vi "GeoData.vi"() -> ()   [LabVIEW 2017] (continued)
17051\tVernon\tIL\tFayette County\tH1\n62418\t17051\tBrownstown\tIL\tFayette County\tH1\n62838\t17051\tFarina\tIL\tFayette County\tH1\n62422\t17051\tCowden\tIL\tFayette County\tH1\n62411\t17051\tAltamont\tIL\tFayette County\tH1\n62875\t17051\tPatoka\tIL\tFayette County\tH1\n62431\t17051\tHerrick\tIL\tFayette County\tH1\n62262\t17051\tMulberry grove\tIL\tFayette County\tH1\n62880\t17051\tSaint peter\tIL\tFayette County\tH1\n62080\t17051\tRamsey\tIL\tFayette County\tH1\n62458\t17051\tSaint elmo\tIL\tFayette County\tH1\n62854\t17051\tKinmundy\tIL\tFayette County\tH1\n60921\t17053\tChatsworth\tIL\tFord County\tH1\n61775\t17053\tStrawn\tIL\tFord County\tH1\n60949\t17053\tLudlow\tIL\tFord County\tH1\n60957\t17053\tPaxton\tIL\tFord County\tH1\n60927\t17053\tClifton\tIL\tFord County\tH1\n60929\t17053\tCullom\tIL\tFord County\tH1\n60946\t17053\tKempton\tIL\tFord County\tH1\n60919\t17053\tCabery\tIL\tFord County\tH1\n60918\t17053\tBuckley\tIL\tFord County\tH1\n60959\t17053\tPiper city\tIL\tFord County\tH1\n60941\t17053\tHerscher\tIL\tFord County\tH1\n60936\t17053\tGibson city\tIL\tFord County\tH1\n60968\t17053\tThawville\tIL\tFord County\tH1\n60955\t17053\tOnarga\tIL\tFord County\tH1\n61773\t17053\tSibley\tIL\tFord County\tH1\n60960\t17053\tRankin\tIL\tFord County\tH1\n60933\t17053\tElliott\tIL\tFord County\tH1\n60917\t17053\tBuckingham\tIL\tFord County\tH1\n60948\t17053\tLoda\tIL\tFord County\tH1\n61840\t17053\tDewey\tIL\tFord County\tH1\n61845\t17053\tFoosland\tIL\tFord County\tH1\n61731\t17053\tCropsey\tIL\tFord County\tH1\n60952\t17053\tMelvin\tIL\tFord County\tH1\n60962\t17053\tRoberts\tIL\tFord County\tH1\n62822\t17055\tChristopher\tIL\tFranklin County\tH1\n62999\t17055\tZeigler\tIL\tFranklin County\tH1\n62810\t17055\tBelle rive\tIL\tFranklin County\tH1\n62932\t17055\tElkville\tIL\tFranklin County\tH1\n62812\t17055\tBenton\tIL\tFranklin County\tH1\n62896\t17055\tWest frankfort\tIL\tFranklin County\tH1\n62860\t17055\tMacedonia\tIL\tFranklin County\tH1\n62836\t17055\tEwing\tIL\tFranklin County\tH1\n62983\t17055\tRoyalton\tIL\tFranklin County\tH1\n62897\t17055\tWhittington\tIL\tFranklin County\tH1\n62891\t17055\tValier\tIL\tFranklin County\tH1\n62840\t17055\tFrankfort heights\tIL\tFranklin County\tH1\n62865\t17055\tMulkeytown\tIL\tFranklin County\tH1\n62890\t17055\tThompsonville\tIL\tFranklin County\tH1\n62884\t17055\tSesser\tIL\tFranklin County\tH1\n62883\t17055\tScheller\tIL\tFranklin County\tH1\n62874\t17055\tOrient\tIL\tFranklin County\tH1\n62825\t17055\tCoello\tIL\tFranklin County\tH1\n62819\t17055\tBuckner\tIL\tFranklin County\tH1\n62856\t17055\tLogan\tIL\tFranklin County\tH1\n61531\t17057\tFarmington\tIL\tFulton County\tH1\n61415\t17057\tAvon\tIL\tFulton County\tH1\n61431\t17057\tEllisville\tIL\tFulton County\tH1\n61544\t17057\tLondon mills\tIL\tFulton County\tH1\n61563\t17057\tSaint david\tIL\tFulton County\tH1\n61520\t17057\tCanton\tIL\tFulton County\tH1\n61459\t17057\tMarietta\tIL\tFulton County\tH1\n61432\t17057\tFairview\tIL\tFulton County\tH1\n61542\t17057\tLewistown\tIL\tFulton County\tH1\n61553\t17057\tNorris\tIL\tFulton County\tH1\n61433\t17057\tFiatt\tIL\tFulton County\tH1\n61427\t17057\tCuba\tIL\tFulton County\tH1\n61569\t17057\tTrivoli\tIL\tFulton County\tH1\n61524\t17057\tDunfermline\tIL\tFulton County\tH1\n61477\t17057\tSmithfield\tIL\tFulton County\tH1\n62644\t17057\tHavana\tIL\tFulton County\tH1\n61482\t17057\tTable grove\tIL\tFulton County\tH1\n61484\t17057\tVermont\tIL\tFulton County\tH1\n61533\t17057\tGlasford\tIL\tFulton County\tH1\n61474\t17057\tSaint augustine\tIL\tFulton County\tH1\n61501\t17057\tAstoria\tIL\tFulton County\tH1\n61519\t17057\tBryant\tIL\tFulton County\tH1\n61441\t17057\tIpava\tIL\tFulton County\tH1\n61543\t17057\tLiverpool\tIL\tFulton County\tH1\n62821\t17059\tCarmi\tIL\tGallatin County\tH1\n62867\t17059\tNew haven\tIL\tGallatin County\tH1\n62984\t17059\tShawneetown\tIL\tGallatin County\tH1\n62930\t17059\tEldorado\tIL\tGallatin County\tH1\n62979\t17059\tRidgway\tIL\tGallatin County\tH1\n62934\t17059\tEquality\tIL\tGallatin County\tH1\n62871\t17059\tOmaha\tIL\tGallatin County\tH1\n62869\t17059\tNorris city\tIL\tGallatin County\tH1\n62954\t17059\tJunction\tIL\tGallatin County\tH1\n62027\t17061\tEldred\tIL\tGreene County\tH1\n62092\t17061\tWhite hall\tIL\tGreene County\tH1\n62054\t17061\tKane\tIL\tGreene County\tH1\n62081\t17061\tRockbridge\tIL\tGreene County\tH1\n62050\t17061\tHillview\tIL\tGreene County\tH1\n62078\t17061\tPatterson\tIL\tGreene County\tH1\n62098\t17061\tWrights\tIL\tGreene County\tH1\n62082\t17061\tRoodhouse\tIL\tGreene County\tH1\n62016\t17061\tCarrollton\tIL\tGreene County\tH1\n62044\t17061\tGreenfield\tIL\tGreene County\tH1\n60424\t17063\tGardner\tIL\tGrundy County\tH1\n60481\t17063\tWilmington\tIL\tGrundy County\tH1\n61360\t17063\tSeneca\tIL\tGrundy County\tH1\n60437\t17063\tKinsman\tIL\tGrundy County\tH1\n60470\t17063\tRansom\tIL\tGrundy County\tH1\n60408\t17063\tBraidwood\tIL\tGrundy County\tH1\n60407\t17063\tBraceville\tIL\tGrundy County\tH1\n60474\t17063\tSouth wilmington\tIL\tGrundy County\tH1\n60410\t17063\tChannahon\tIL\tGrundy County\tH1\n60479\t17063\tVerona\tIL\tGrundy County\tH1\n60961\t17063\tReddick\tIL\tGrundy County\tH1\n60447\t17063\tMinooka\tIL\tGrundy County\tH1\n60444\t17063\tMazon\tIL\tGrundy County\tH1\n60416\t17063\tCoal city\tIL\tGrundy County\tH1\n60420\t17063\tDwight\tIL\tGrundy County\tH1\n60541\t17063\tNewark\tIL\tGrundy County\tH1\n60450\t17063\tMorris\tIL\tGrundy County\tH1\n62828\t17065\tDahlgren\tIL\tHamilton County\tH1\n62810\t17065\tBelle rive\tIL\tHamilton County\tH1\n62835\t17065\tEnfield\tIL\tHamilton County\tH1\n62860\t17065\tMacedonia\tIL\tHamilton County\tH1\n62930\t17065\tEldorado\tIL\tHamilton County\tH1\n62817\t17065\tBroughton\tIL\tHamilton County\tH1\n62829\t17065\tDale\tIL\tHamilton County\tH1\n62887\t17065\tSpringerton\tIL\tHamilton County\tH1\n62859\t17065\tMc leansboro\tIL\tHamilton County\tH1\n62935\t17065\tGalatia\tIL\tHamilton County\tH1\n62379\t17067\tWarsaw\tIL\tHancock County\tH1\n62326\t17067\tColchester\tIL\tHancock County\tH1\n62316\t17067\tBowen\tIL\tHancock County\tH1\n62330\t17067\tDallas city\tIL\tHancock County\tH1\n62374\t17067\tTennessee\tIL\tHancock County\tH1\n61450\t17067\tLa harpe\tIL\tHancock County\tH1\n62351\t17067\tMendon\tIL\tHancock County\tH1\n62313\t17067\tBasco\tIL\tHancock County\tH1\n62380\t17067\tWest point\tIL\tHancock County\tH1\n62334\t17067\tElvaston\tIL\tHancock County\tH1\n62341\t17067\tHamilton\tIL\tHancock County\tH1\n62373\t17067\tSutter\tIL\tHancock County\tH1\n62329\t17067\tColusa\tIL\tHancock County\tH1\n61420\t17067\tBlandinsville\tIL\tHancock County\tH1\n62346\t17067\tLa prairie\tIL\tHancock County\tH1\n62321\t17067\tCarthage\tIL\tHancock County\tH1\n62311\t17067\tAugusta\tIL\tHancock County\tH1\n62336\t17067\tFerris\tIL\tHancock County\tH1\n62354\t17067\tNauvoo\tIL\tHancock County\tH1\n62349\t17067\tLoraine\tIL\tHancock County\tH1\n62367\t17067\tPlymouth\tIL\tHancock County\tH1\n62358\t17067\tNiota\tIL\tHancock County\tH1\n62947\t17069\tHerod\tIL\tHardin County\tH1\n62955\t17069\tKarbers ridge\tIL\tHardin County\tH1\n62931\t17069\tElizabethtown\tIL\tHardin County\tH1\n62919\t17069\tCave in rock\tIL\tHardin County\tH1\n62982\t17069\tRosiclare\tIL\tHardin County\tH1\n61418\t17071\tBiggsville\tIL\tHenderson County\tH1\n61460\t17071\tMedia\tIL\tHenderson County\tH1\n62330\t17071\tDallas city\tIL\tHenderson County\tH1\n61454\t17071\tLomax\tIL\tHenderson County\tH1\n61450\t17071\tLa harpe\tIL\tHenderson County\tH1\n61469\t17071\tOquawka\tIL\tHenderson County\tH1\n61471\t17071\tRaritan\tIL\tHenderson County\tH1\n61480\t17071\tStronghurst\tIL\tHenderson County\tH1\n61437\t17071\tGladstone\tIL\tHenderson County\tH1\n61425\t17071\tCarman\tIL\tHenderson County\tH1\n61254\t17073\tGeneseo\tIL\tHenry County\tH1\n61235\t17073\tAtkinson\tIL\tHenry County\tH1\n61233\t17073\tAndover\tIL\tHenry County\tH1\n61240\t17073\tCoal valley\tIL\tHenry County\tH1\n61443\t17073\tKewanee\tIL\tHenry County\tH1\n61344\t17073\tMineral\tIL\tHenry County\tH1\n61241\t17073\tColona\tIL\tHenry County\tH1\n61283\t17073\tTampico\tIL\tHenry County\tH1\n61465\t17073\tNew windsor\tIL\tHenry County\tH1\n61262\t17073\tLynn center\tIL\tHenry County\tH1\n61258\t17073\tHooppole\tIL\tHenry County\tH1\n61238\t17073\tCambridge\tIL\tHenry County\tH1\n61274\t17073\tOsco\tIL\tHenry County\tH1\n61413\t17073\tAlpha\tIL\tHenry County\tH1\n61468\t17073\tOphiem\tIL\tHenry County\tH1\n61490\t17073\tWoodhull\tIL\tHenry County\tH1\n61361\t17073\tSheffield\tIL\tHenry County\tH1\n61419\t17073\tBishop hill\tIL\tHenry County\tH1\n61234\t17073\tAnnawan\tIL\tHenry County\tH1\n61273\t17073\tOrion\tIL\tHenry County\tH1\n61277\t17073\tProphetstown\tIL\tHenry County\tH1\n61250\t17073\tErie\tIL\tHenry County\tH1\n61434\t17073\tGalva\tIL\tHenry County\tH1\n61414\t17073\tAltona\tIL\tHenry County\tH1\n60912\t17075\tBeaverville\tIL\tIroquois County\tH1\n60964\t17075\tSaint anne\tIL\tIroquois County\tH1\n60928\t17075\tCrescent city\tIL\tIroquois County\tH1\n60951\t17075\tMartinton\tIL\tIroquois County\tH1\n60931\t17075\tDonovan\tIL\tIroquois County\tH1\n60939\t17075\tGoodwine\tIL\tIroquois County\tH1\n60927\t17075\tClifton\tIL\tIroquois County\tH1\n60973\t17075\tWellington\tIL\tIroquois County\tH1\n60974\t17075\tWoodland\tIL\tIroquois County\tH1\n60918\t17075\tBuckley\tIL\tIroquois County\tH1\n60956\t17075\tPapineau\tIL\tIroquois County\tH1\n60941\t17075\tHerscher\tIL\tIroquois County\tH1\n60970\t17075\tWatseka\tIL\tIroquois County\tH1\n60966\t17075\tSheldon\tIL\tIroquois County\tH1\n60968\t17075\tThawville\tIL\tIroquois County\tH1\n60955\t17075\tOnarga\tIL\tIroquois County\tH1\n60924\t17075\tCissna park\tIL\tIroquois County\tH1\n60967\t17075\tStockland\tIL\tIroquois County\tH1\n60911\t17075\tAshkum\tIL\tIroquois County\tH1\n60960\t17075\tRankin\tIL\tIroquois County\tH1\n60938\t17075\tGilman\tIL\tIroquois County\tH1\n60953\t17075\tMilford\tIL\tIroquois County\tH1\n60945\t17075\tIroquois\tIL\tIroquois County\tH1\n60926\t17075\tClaytonville\tIL\tIroquois County\tH1\n60930\t17075\tDanforth\tIL\tIroquois County\tH1\n60948\t17075\tLoda\tIL\tIroquois County\tH1\n60942\t17075\tHoopeston\tIL\tIroquois County\tH1\n60922\t17075\tChebanse\tIL\tIroquois County\tH1\n62272\t17077\tPercy\tIL\tJackson County\tH1\n62918\t17077\tCarterville\tIL\tJackson County\tH1\n62975\t17077\tPomona\tIL\tJackson County\tH1\n62932\t17077\tElkville\tIL\tJackson County\tH1\n62942\t17077\tGrand tower\tIL\tJackson County\tH1\n62905\t17077\tAlto pass\tIL\tJackson County\tH1\n62958\t17077\tMakanda\tIL\tJackson County\tH1\n62907\t17077\tAva\tIL\tJackson County\tH1\n62924\t17077\tDe soto\tIL\tJackson County\tH1\n62916\t17077\tCampbell hill\tIL\tJackson County\tH1\n62927\t17077\tDowell\tIL\tJackson County\tH1\n62940\t17077\tGorham\tIL\tJackson County\tH1\n62994\t17077\tVergennes\tIL\tJackson County\tH1\n62950\t17077\tJacob\tIL\tJackson County\tH1\n62901\t17077\tCarbondale\tIL\tJackson County\tH1\n62903\t17077\tCarbondale\tIL\tJackson County\tH1\n62280\t17077\tRockwood\tIL\tJackson County\tH1\n62832\t17077\tDu quoin\tIL\tJackson County\tH1\n62966\t17077\tMurphysboro\tIL\tJackson County\tH1\n62920\t17077\tCobden\tIL\tJackson County\tH1\n62902\t17077\tCarbondale\tIL\tJackson County\tH1\n62448\t17079\tNewton\tIL\tJasper County\tH1\n62479\t17079\tWheeler\tIL\tJasper County\tH1\n62445\t17079\tMontrose\tIL\tJasper County\tH1\n62420\t17079\tCasey\tIL\tJasper County\tH1\n62428\t17079\tGreenup\tIL\tJasper County\tH1\n62425\t17079\tDundas\tIL\tJasper County\tH1\n62481\t17079\tYale\tIL\tJasper County\tH1\n62424\t17079\tDieterich\tIL\tJasper County\tH1\n62432\t17079\tHidalgo\tIL\tJasper County\tH1\n62475\t17079\tWest liberty\tIL\tJasper County\tH1\n62480\t17079\tWillow hill\tIL\tJasper County\tH1\n62436\t17079\tJewett\tIL\tJasper County\tH1\n62459\t17079\tSainte marie\tIL\tJasper County\tH1\n62467\t17079\tTeutopolis\tIL\tJasper County\tH1\n62449\t17079\tOblong\tIL\tJasper County\tH1\n62434\t17079\tIngraham\tIL\tJasper County\tH1\n62864\t17081\tMount vernon\tIL\tJefferson County\tH1\n62872\t17081\tOpdyke\tIL\tJefferson County\tH1\n62828\t17081\tDahlgren\tIL\tJefferson County\tH1\n62810\t17081\tBelle rive\tIL\tJefferson County\tH1\n62851\t17081\tKeenes\tIL\tJefferson County\tH1\n62894\t17081\tWaltonville\tIL\tJefferson County\tH1\n62830\t17081\tDix\tIL\tJefferson County\tH1\n62801\t17081\tCentralia\tIL\tJefferson County\tH1\n62808\t17081\tAshley\tIL\tJefferson County\tH1\n62889\t17081\tTexico\tIL\tJefferson County\tH1\n62860\t17081\tMacedonia\tIL\tJefferson County\tH1\n62816\t17081\tBonnie\tIL\tJefferson County\tH1\n62846\t17081\tIna\tIL\tJefferson County\tH1\n62836\t17081\tEwing\tIL\tJefferson County\tH1\n62893\t17081\tWalnut hill\tIL\tJefferson County\tH1\n62814\t17081\tBluford\tIL\tJefferson County\tH1\n62831\t17081\tDu bois\tIL\tJefferson County\tH1\n62853\t17081\tKell\tIL\tJefferson County\tH1\n62884\t17081\tSesser\tIL\tJefferson County\tH1\n62898\t17081\tWoodlawn\tIL\tJefferson County\tH1\n62883\t17081\tScheller\tIL\tJefferson County\tH1\n62877\t17081\tRichview\tIL\tJefferson County\tH1\n62035\t17083\tGodfrey\tIL\tJersey County\tH1\n62031\t17083\tFieldon\tIL\tJersey County\tH1\n62054\t17083\tKane\tIL\tJersey County\tH1\n62030\t17083\tFidelity\tIL\tJersey County\tH1\n62028\t17083\tElsah\tIL\tJersey County\tH1\n62012\t17083\tBrighton\tIL\tJersey County\tH1\n62052\t17083\tJerseyville\tIL\tJersey County\tH1\n62065\t17083\tMichael\tIL\tJersey County\tH1\n62079\t17083\tPiasa\tIL\tJersey County\tH1\n62037\t17083\tGrafton\tIL\tJersey County\tH1\n62022\t17083\tDow\tIL\tJersey County\tH1\n62063\t17083\tMedora\tIL\tJersey County\tH1\n61085\t17085\tStockton\tIL\tJo Daviess County\tH1\n61036\t17085\tGalena\tIL\tJo Daviess County\tH1\n61053\t17085\tMount carroll\tIL\tJo Daviess County\tH1\n61087\t17085\tWarren\tIL\tJo Daviess County\tH1\n61089\t17085\tWinslow\tIL\tJo Daviess County\tH1\n61062\t17085\tPearl city\tIL\tJo Daviess County\tH1\n61048\t17085\tLena\tIL\tJo Daviess County\tH1\n61044\t17085\tKent\tIL\tJo Daviess County\tH1\n61001\t17085\tApple river\tIL\tJo Daviess County\tH1\n61025\t17085\tEast dubuque\tIL\tJo Daviess County\tH1\n61028\t17085\tElizabeth\tIL\tJo Daviess County\tH1\n61074\t17085\tSavanna\tIL\tJo Daviess County\tH1\n61075\t17085\tScales mound\tIL\tJo Daviess County\tH1\n61059\t17085\tNora\tIL\tJo Daviess County\tH1\n61041\t17085\tHanover\tIL\tJo Daviess County\tH1\n62972\t17087\tOzark\tIL\tJohnson County\tH1\n62985\t17087\tSimpson\tIL\tJohnson County\tH1\n62943\t17087\tGrantsburg\tIL\tJohnson County\tH1\n62938\t17087\tGolconda\tIL\tJohnson County\tH1\n62912\t17087\tBuncombe\tIL\tJohnson County\tH1\n62908\t17087\tBelknap\tIL\tJohnson County\tH1\n62939\t17087\tGoreville\tIL\tJohnson County\tH1\n62922\t17087\tCreal springs\tIL\tJohnson County\tH1\n62909\t17087\tBoles\tIL\tJohnson County\tH1\n62967\t17087\tNew burnside\tIL\tJohnson County\tH1\n62995\t17087\tVienna\tIL\tJohnson County\tH1\n62902\t17087\tCarbondale\tIL\tJohnson County\tH1\n62923\t17087\tCypress\tIL\tJohnson County\tH1\n60136\t17089\tGilberts\tIL\tKane County\tH1\n60144\t17089\tKaneville\tIL\tKane County\tH1\n60192\t17089\tHoffman estates\tIL\tKane County\tH1\n60175\t17089\tSaint charles\tIL\tKane County\tH1\n60502\t17089\tAurora\tIL\tKane County\tH1\n60178\t17089\tSycamore\tIL\tKane County\tH1\n60507\t17089\tAurora\tIL\tKane County\tH1\n60503\t17089\tAurora\tIL\tKane County\tH1\n60103\t17089\tBartlett\tIL\tKane County\tH1\n60110\t17089\tCarpentersville\tIL\tKane County\tH1\n60102\t17089\tAlgonquin\tIL\tKane County\tH1\n60142\t17089\tHuntley\tIL\tKane County\tH1\n60177\t17089\tSouth elgin\tIL\tKane County\tH1\n60123\t17089\tElgin\tIL\tKane County\tH1\n60124\t17089\tElgin\tIL\tKane County\tH1\n60543\t17089\tOswego\tIL\tKane County\tH1\n60538\t17089\tMontgomery\tIL\tKane County\tH1\n60121\t17089\tElgin\tIL\tKane County\tH1\n60184\t17089\tWayne\tIL\tKane County\tH1\n60510\t17089\tBatavia\tIL\tKane County\tH1\n60511\t17089\tBig rock\tIL\tKane County\tH1\n60120\t17089\tElgin\tIL\tKane County\tH1\n60119\t17089\tElburn\tIL\tKane County\tH1\n60542\t17089\tNorth aurora\tIL\tKane County\tH1\n60545\t17089\tPlano\tIL\tKane County\tH1\n60010\t17089\tBarrington\tIL\tKane County\tH1\n60185\t17089\tWest chicago\tIL\tKane County\tH1\n60506\t17089\tAurora\tIL\tKane County\tH1\n60134\t17089\tGeneva\tIL\tKane County\tH1\n60147\t17089\tLafox\tIL\tKane County\tH1\n60520\t17089\tHinckley\tIL\tKane County\tH1\n60135\t17089\tGenoa\tIL\tKane County\tH1\n60109\t17089\tBurlington\tIL\tKane County\tH1\n60183\t17089\tWasco\tIL\tKane County\tH1\n60174\t17089\tSaint charles\tIL\tKane County\tH1\n60504\t17089\tAurora\tIL\tKane County\tH1\n60505\t17089\tAurora\tIL\tKane County\tH1\n60140\t17089\tHampshire\tIL\tKane County\tH1\n60118\t17089\tDundee\tIL\tKane County\tH1\n60151\t17089\tMaple park\tIL\tKane County\tH1\n60554\t17089\tSugar grove\tIL\tKane County\tH1\n60539\t17089\tMooseheart\tIL\tKane County\tH1\n60424\t17091\tGardner\tIL\tKankakee County\tH1\n60481\t17091\tWilmington\tIL\tKankakee County\tH1\n60964\t17091\tSaint anne\tIL\tKankakee County\tH1\n60969\t17091\tUnion hill\tIL\tKankakee County\tH1\n60914\t17091\tBourbonnais\tIL\tKankakee County\tH1\n60954\t17091\tMomence\tIL\tKankakee County\tH1\n60935\t17091\tEssex\tIL\tKankakee County\tH1\n60919\t17091\tCabery\tIL\tKankakee County\tH1\n60401\t17091\tBeecher\tIL\tKankakee County\tH1\n60901\t17091\tKankakee\tIL\tKankakee County\tH1\n60915\t17091\tBradley\tIL\tKankakee County\tH1\n60941\t17091\tHerscher\tIL\tKankakee County\tH1\n60950\t17091\tManteno\tIL\tKankakee County\tH1\n60958\t17091\tPembroke township\tIL\tKankakee County\tH1\n60961\t17091\tReddick\tIL\tKankakee County\tH1\n60944\t17091\tHopkins park\tIL\tKankakee County\tH1\n60910\t17091\tAroma park\tIL\tKankakee County\tH1\n60917\t17091\tBuckingham\tIL\tKankakee County\tH1\n60468\t17091\tPeotone\tIL\tKankakee County\tH1\n60940\t17091\tGrant park\tIL\tKankakee County\tH1\n60922\t17091\tChebanse\tIL\tKankakee County\tH1\n60913\t17091\tBonfield\tIL\tKankakee County\tH1\n60544\t17093\tPlainfield\tIL\tKendall County\tH1\n60548\t17093\tSandwich\tIL\tKendall County\tH1\n60585\t17093\tPlainfield\tIL\tKendall County\tH1\n60431\t17093\tJoliet\tIL\tKendall County\tH1\n60503\t17093\tAurora\tIL\tKendall County\tH1\n60512\t17093\tBristol\tIL\tKendall County\tH1\n60435\t17093\tJoliet\tIL\tKendall County\tH1\n60543\t17093\tOswego\tIL\tKendall County\tH1\n60538\t17093\tMontgomery\tIL\tKendall County\tH1\n60560\t17093\tYorkville\tIL\tKendall County\tH1\n60447\t17093\tMinooka\tIL\tKendall County\tH1\n60511\t17093\tBig rock\tIL\tKendall County\tH1\n60545\t17093\tPlano\tIL\tKendall County\tH1\n60506\t17093\tAurora\tIL\tKendall County\tH1\n60586\t17093\tPlainfield\tIL\tKendall County\tH1\n60541\t17093\tNewark\tIL\tKendall County\tH1\n60536\t17093\tMillbrook\tIL\tKendall County\tH1\n60537\t17093\tMillington\tIL\tKendall County\tH1\n60551\t17093\tSheridan\tIL\tKendall County\tH1\n60450\t17093\tMorris\tIL\tKendall County\tH1\n60504\t17093\tAurora\tIL\tKendall County\tH1\n60554\t17093\tSugar grove\tIL\tKendall County\tH1\n61412\t17095\tAlexis\tIL\tKnox County\tH1\n61529\t17095\tElmwood\tIL\tKnox County\tH1\n61531\t17095\tFarmington\tIL\tKnox County\tH1\n61458\t17095\tMaquon\tIL\tKnox County\tH1\n61449\t17095\tLa fayette\tIL\tKnox County\tH1\n61544\t17095\tLondon mills\tIL\tKnox County\tH1\n61448\t17095\tKnoxville\tIL\tKnox County\tH1\n61410\t17095\tAbingdon\tIL\tKnox County\tH1\n61467\t17095\tOneida\tIL\tKnox County\tH1\n61423\t17095\tCameron\tIL\tKnox County\tH1\n61439\t17095\tHenderson\tIL\tKnox County\tH1\n61401\t17095\tGalesburg\tIL\tKnox County\tH1\n61472\t17095\tRio\tIL\tKnox County\tH1\n61428\t17095\tDahinda\tIL\tKnox County\tH1\n61485\t17095\tVictoria\tIL\tKnox County\tH1\n61490\t17095\tWoodhull\tIL\tKnox County\tH1\n61466\t17095\tNorth henderson\tIL\tKnox County\tH1\n61488\t17095\tWataga\tIL\tKnox County\tH1\n61572\t17095\tYates city\tIL\tKnox County\tH1\n61430\t17095\tEast galesburg\tIL\tKnox County\tH1\n61434\t17095\tGalva\tIL\tKnox County\tH1\n61414\t17095\tAltona\tIL\tKnox County\tH1\n61474\t17095\tSaint augustine\tIL\tKnox County\tH1\n61489\t17095\tWilliamsfield\tIL\tKnox County\tH1\n61436\t17095\tGilson\tIL\tKnox County\tH1\n61402\t17095\tGalesburg\tIL\tKnox County\tH1\n60051\t17097\tMchenry\tIL\tLake County\tH1\n60067\t17097\tPalatine\tIL\tLake County\tH1\n60047\t17097\tLake zurich\tIL\tLake County\tH1\n60050\t17097\tMchenry\tIL\tLake County\tH1\n60042\t17097\tIsland lake\tIL\tLake County\tH1\n60069\t17097\tLincolnshire\tIL\tLake County\tH1\n60090\t17097\tWheeling\tIL\tLake County\tH1\n60089\t17097\tBuffalo grove\tIL\tLake County\tH1\n60013\t17097\tCary\tIL\tLake County\tH1\n60045\t17097\tLake forest\tIL\tLake County\tH1\n60011\t17097\tBarrington\tIL\tLake County\tH1\n60021\t17097\tFox river grove\tIL\tLake County\tH1\n60037\t17097\tFort sheridan\tIL\tLake County\tH1\n60061\t17097\tVernon hills\tIL\tLake County\tH1\n60079\t17097\tWaukegan\tIL\tLake County\tH1\n60002\t17097\tAntioch\tIL\tLake County\tH1\n60073\t17097\tRound lake\tIL\tLake County\tH1\n60084\t17097\tWauconda\tIL\tLake County\tH1\n60088\t17097\tGreat lakes\tIL\tLake County\tH1\n60060\t17097\tMundelein\tIL\tLake County\tH1\n60096\t17097\tWinthrop harbor\tIL\tLake County\tH1\n60015\t17097\tDeerfield\tIL\tLake County\tH1\n60075\t17097\tRussell\tIL\tLake County\tH1\n60085\t17097\tWaukegan\tIL\tLake County\tH1\n60087\t17097\tWaukegan\tIL\tLake County\tH1\n60081\t17097\tSpring grove\tIL\tLake County\tH1\n60099\t17097\tZion\tIL\tLake County\tH1\n60035\t17097\tHighland park\tIL\tLake County\tH1\n60040\t17097\tHighwood\tIL\tLake County\tH1\n60083\t17097\tWadsworth\tIL\tLake County\tH1\n60010\t17097\tBarrington\tIL\tLake County\tH1\n60031\t17097\tGurnee\tIL\tLake County\tH1\n60044\t17097\tLake bluff\tIL\tLake County\tH1\n60074\t17097\tPalatine\tIL\tLake County\tH1\n60064\t17097\tNorth chicago\tIL\tLake County\tH1\n60020\t17097\tFox lake\tIL\tLake County\tH1\n60030\t17097\tGrayslake\tIL\tLake County\tH1\n60046\t17097\tLake villa\tIL\tLake County\tH1\n60048\t17097\tLibertyville\tIL\tLake County\tH1\n60041\t17097\tIngleside\tIL\tLake County\tH1\n60086\t17097\tNorth chicago\tIL\tLake County\tH1\n61360\t17099\tSeneca\tIL\tLaSalle County\tH1\n60437\t17099\tKinsman\tIL\tLaSalle County\tH1\n60552\t17099\tSomonauk\tIL\tLaSalle County\tH1\n60548\t17099\tSandwich\tIL\tLaSalle County\tH1\n60549\t17099\tSerena\tIL\tLaSalle County\tH1\n61373\t17099\tUtica\tIL\tLaSalle County\tH1\n61311\t17099\tAncona\tIL\tLaSalle County\tH1\n61358\t17099\tRutland\tIL\tLaSalle County\tH1\n60470\t17099\tRansom\tIL\tLaSalle County\tH1\n60531\t17099\tLeland\tIL\tLaSalle County\tH1\n61377\t17099\tWenona\tIL\tLaSalle County\tH1\n61301\t17099\tLa salle\tIL\tLaSalle County\tH1\n61342\t17099\tMendota\tIL\tLaSalle County\tH1\n60557\t17099\tWedron\tIL\tLaSalle County\tH1\n61372\t17099\tTroy grove\tIL\tLaSalle County\tH1\n61354\t17099\tPeru\tIL\tLaSalle County\tH1\n61370\t17099\tTonica\tIL\tLaSalle County\tH1\n61336\t17099\tMagnolia\tIL\tLaSalle County\tH1\n60541\t17099\tNewark\tIL\tLaSalle County\tH1\n61348\t17099\tOglesby\tIL\tLaSalle County\tH1\n61350\t17099\tOttawa\tIL\tLaSalle County\tH1\n61334\t17099\tLostant\tIL\tLaSalle County\tH1\n61333\t17099\tLong point\tIL\tLaSalle County\tH1\n61320\t17099\tDalzell\tIL\tLaSalle County\tH1\n60537\t17099\tMillington\tIL\tLaSalle County\tH1\n60551\t17099\tSheridan\tIL\tLaSalle County\tH1\n61364\t17099\tStreator\tIL\tLaSalle County\tH1\n61325\t17099\tGrand ridge\tIL\tLaSalle County\tH1\n61321\t17099\tDana\tIL\tLaSalle County\tH1\n61332\t17099\tLeonore\tIL\tLaSalle County\tH1\n61316\t17099\tCedar point\tIL\tLaSalle County\tH1\n60518\t17099\tEarlville\tIL\tLaSalle County\tH1\n61341\t17099\tMarseilles\tIL\tLaSalle County\tH1\n61371\t17099\tTriumph\tIL\tLaSalle County\tH1\n62439\t17101\tLawrenceville\tIL\tLawrence County\tH1\n62410\t17101\tAllendale\tIL\tLawrence County\tH1\n62466\t17101\tSumner\tIL\tLawrence County\tH1\n62460\t17101\tSaint francisville\tIL\tLawrence County\tH1\n62427\t17101\tFlat rock\tIL\tLawrence County\tH1\n62417\t17101\tBridgeport\tIL\tLawrence County\tH1\n60553\t17103\tSteward\tIL\tLee County\tH1\n61006\t17103\tAshton\tIL\tLee County\tH1\n61349\t17103\tOhio\tIL\tLee County\tH1\n61318\t17103\tCompton\tIL\tLee County\tH1\n61068\t17103\tRochelle\tIL\tLee County\tH1\n61342\t17103\tMendota\tIL\tLee County\tH1\n61353\t17103\tPaw paw\tIL\tLee County\tH1\n61042\t17103\tHarmon\tIL\tLee County\tH1\n61057\t17103\tNachusa\tIL\tLee County\tH1\n61064\t17103\tPolo\tIL\tLee County\tH1\n61243\t17103\tDeer grove\tIL\tLee County\tH1\n61081\t17103\tSterling\tIL\tLee County\tH1\n61376\t17103\tWalnut\tIL\tLee County\tH1\n61031\t17103\tFranklin grove\tIL\tLee County\tH1\n61331\t17103\tLee center\tIL\tLee County\tH1\n60530\t17103\tLee\tIL\tLee County\tH1\n61378\t17103\tWest brooklyn\tIL\tLee County\tH1\n61367\t17103\tSublette\tIL\tLee County\tH1\n61330\t17103\tLa moille\tIL\tLee County\tH1\n61324\t17103\tEldena\tIL\tLee County\tH1\n61071\t17103\tRock falls\tIL\tLee County\tH1\n61021\t17103\tDixon\tIL\tLee County\tH1\n60518\t17103\tEarlville\tIL\tLee County\tH1\n61310\t17103\tAmboy\tIL\tLee County\tH1\n60921\t17105\tChatsworth\tIL\tLivingston County\tH1\n61744\t17105\tGridley\tIL\tLivingston County\tH1\n61775\t17105\tStrawn\tIL\tLivingston County\tH1\n60929\t17105\tCullom\tIL\tLivingston County\tH1\n61311\t17105\tAncona\tIL\tLivingston County\tH1\n61739\t17105\tFairbury\tIL\tLivingston County\tH1\n60470\t17105\tRansom\tIL\tLivingston County\tH1\n60946\t17105\tKempton\tIL\tLivingston County\tH1\n60919\t17105\tCabery\tIL\tLivingston County\tH1\n60959\t17105\tPiper city\tIL\tLivingston County\tH1\n60460\t17105\tOdell\tIL\tLivingston County\tH1\n60961\t17105\tReddick\tIL\tLivingston County\tH1\n61726\t17105\tChenoa\tIL\tLivingston County\tH1\n61728\t17105\tColfax\tIL\tLivingston County\tH1\n60934\t17105\tEmington\tIL\tLivingston County\tH1\n61319\t17105\tCornell\tIL\tLivingston County\tH1\n61743\t17105\tGraymont\tIL\tLivingston County\tH1\n61313\t17105\tBlackstone\tIL\tLivingston County\tH1\n60420\t17105\tDwight\tIL\tLivingston County\tH1\n60917\t17105\tBuckingham\tIL\tLivingston County\tH1\n61333\t17105\tLong point\tIL\tLivingston County\tH1\n61769\t17105\tSaunemin\tIL\tLivingston County\tH1\n61364\t17105\tStreator\tIL\tLivingston County\tH1\n61764\t17105\tPontiac\tIL\tLivingston County\tH1\n61741\t17105\tForrest\tIL\tLivingston County\tH1\n61740\t17105\tFlanagan\tIL\tLivingston County\tH1\n61731\t17105\tCropsey\tIL\tLivingston County\tH1\n60920\t17105\tCampus\tIL\tLivingston County\tH1\n61760\t17105\tMinonk\tIL\tLivingston County\tH1\n60952\t17105\tMelvin\tIL\tLivingston County\tH1\n60962\t17105\tRoberts\tIL\tLivingston County\tH1\n62634\t17107\tElkhart\tIL\tLogan County\tH1\n61723\t17107\tAtlanta\tIL\tLogan County\tH1\n62518\t17107\tChestnut\tIL\tLogan County\tH1\n62519\t17107\tCornland\tIL\tLogan County\tH1\n62548\t17107\tMount pulaski\tIL\tLogan County\tH1\n62656\t17107\tLincoln\tIL\tLogan County\tH1\n62671\t17107\tNew holland\tIL\tLogan County\tH1\n61754\t17107\tMc lean\tIL\tLogan County\tH1\n62682\t17107\tSan jose\tIL\tLogan County\tH1\n61751\t17107\tLawndale\tIL\tLogan County\tH1\n62635\t17107\tEmden\tIL\tLogan County\tH1\n62693\t17107\tWilliamsville\tIL\tLogan County\tH1\n62613\t17107\tAthens\tIL\tLogan County\tH1\n61749\t17107\tKenney\tIL\tLogan County\tH1\n62666\t17107\tMiddletown\tIL\tLogan County\tH1\n62541\t17107\tLake fork\tIL\tLogan County\tH1\n62543\t17107\tLatham\tIL\tLogan County\tH1\n61721\t17107\tArmington\tIL\tLogan County\tH1\n62512\t17107\tBeason\tIL\tLogan County\tH1\n62643\t17107\tHartsburg\tIL\tLogan County\tH1\n61440\t17109\tIndustry\tIL\tMcDonough County\tH1\n61415\t17109\tAvon\tIL\tMcDonough County\tH1\n61475\t17109\tSciota\tIL\tMcDonough County\tH1\n61452\t17109\tLittleton\tIL\tMcDonough County\tH1\n62326\t17109\tColchester\tIL\tMcDonough County\tH1\n61459\t17109\tMarietta\tIL\tMcDonough County\tH1\n62374\t17109\tTennessee\tIL\tMcDonough County\tH1\n61470\t17109\tPrairie city\tIL\tMcDonough County\tH1\n61450\t17109\tLa harpe\tIL\tMcDonough County\tH1\n61473\t17109\tRoseville\tIL\tMcDonough County\tH1\n61455\t17109\tMacomb\tIL\tMcDonough County\tH1\n61438\t17109\tGood hope\tIL\tMcDonough County\tH1\n61422\t17109\tBushnell\tIL\tMcDonough County\tH1\n61411\t17109\tAdair\tIL\tMcDonough County\tH1\n61420\t17109\tBlandinsville\tIL\tMcDonough County\tH1\n61482\t17109\tTable grove\tIL\tMcDonough County\tH1\n61484\t17109\tVermont\tIL\tMcDonough County\tH1\n62367\t17109\tPlymouth\tIL\tMcDonough County\tH1\n61416\t17109\tBardolph\tIL\tMcDonough County\tH1\n60051\t17111\tMchenry\tIL\tMcHenry County\tH1\n60067\t17111\tPalatine\tIL\tMcHenry County\tH1\n60098\t17111\tWoodstock\tIL\tMcHenry County\tH1\n60050\t17111\tMchenry\tIL\tMcHenry County\tH1\n60042\t17111\tIsland lake\tIL\tMcHenry County\tH1\n60152\t17111\tMarengo\tIL\tMcHenry County\tH1\n61012\t17111\tCapron\tIL\tMcHenry County\tH1\n60013\t17111\tCary\tIL\tMcHenry County\tH1\n60021\t17111\tFox river grove\tIL\tMcHenry County\tH1\n60071\t17111\tRichmond\tIL\tMcHenry County\tH1\n60002\t17111\tAntioch\tIL\tMcHenry County\tH1\n60102\t17111\tAlgonquin\tIL\tMcHenry County\tH1\n60142\t17111\tHuntley\tIL\tMcHenry County\tH1\n60072\t17111\tRingwood\tIL\tMcHenry County\tH1\n61038\t17111\tGarden prairie\tIL\tMcHenry County\tH1\n60097\t17111\tWonder lake\tIL\tMcHenry County\tH1\n60081\t17111\tSpring grove\tIL\tMcHenry County\tH1\n60033\t17111\tHarvard\tIL\tMcHenry County\tH1\n60010\t17111\tBarrington\tIL\tMcHenry County\tH1\n60014\t17111\tCrystal lake\tIL\tMcHenry County\tH1\n60156\t17111\tLake in the hills\tIL\tMcHenry County\tH1\n60039\t17111\tCrystal lake\tIL\tMcHenry County\tH1\n60020\t17111\tFox lake\tIL\tMcHenry County\tH1\n60034\t17111\tHebron\tIL\tMcHenry County\tH1\n60135\t17111\tGenoa\tIL\tMcHenry County\tH1\n60012\t17111\tCrystal lake\tIL\tMcHenry County\tH1\n60140\t17111\tHampshire\tIL\tMcHenry County\tH1\n60180\t17111\tUnion\tIL\tMcHenry County\tH1\n61723\t17113\tAtlanta\tIL\tMcLean County\tH1\n61761\t17113\tNormal\tIL\tMcLean County\tH1\n61744\t17113\tGridley\tIL\tMcLean County\tH1\n61745\t17113\tHeyworth\tIL\tMcLean County\tH1\n61770\t17113\tSaybrook\tIL\tMcLean County\tH1\n61776\t17113\tTowanda\tIL\tMcLean County\tH1\n61799\t17113\tBloomington\tIL\tMcLean County\tH1\n61739\t17113\tFairbury\tIL\tMcLean County\tH1\n61732\t17113\tDanvers\tIL\tMcLean County\tH1\n61772\t17113\tShirley\tIL\tMcLean County\tH1\n61759\t17113\tMinier\tIL\tMcLean County\tH1\n61758\t17113\tMerna\tIL\tMcLean County\tH1\n61737\t17113\tEllsworth\tIL\tMcLean County\tH1\n61774\t17113\tStanford\tIL\tMcLean County\tH1\n61724\t17113\tBellflower\tIL\tMcLean County\tH1\n61843\t17113\tFisher\tIL\tMcLean County\tH1\n61790\t17113\tNormal\tIL\tMcLean County\tH1\n60936\t17113\tGibson city\tIL\tMcLean County\tH1\n61701\t17113\tBloomington\tIL\tMcLean County\tH1\n61726\t17113\tChenoa\tIL\tMcLean County\tH1\n61728\t17113\tColfax\tIL\tMcLean County\tH1\n61754\t17113\tMc lean\tIL\tMcLean County\tH1\n61702\t17113\tBloomington\tIL\tMcLean County\tH1\n61722\t17113\tArrowsmith\tIL\tMcLean County\tH1\n61755\t17113\tMackinaw\tIL\tMcLean County\tH1\n61842\t17113\tFarmer city\tIL\tMcLean County\tH1\n61854\t17113\tMansfield\tIL\tMcLean County\tH1\n61725\t17113\tCarlock\tIL\tMcLean County\tH1\n61748\t17113\tHudson\tIL\tMcLean County\tH1\n61752\t17113\tLe roy\tIL\tMcLean County\tH1\n61753\t17113\tLexington\tIL\tMcLean County\tH1\n61730\t17113\tCooksville\tIL\tMcLean County\tH1\n61729\t17113\tCongerville\tIL\tMcLean County\tH1\n61791\t17113\tBloomington\tIL\tMcLean County\tH1\n61705\t17113\tBloomington\tIL\tMcLean County\tH1\n61720\t17113\tAnchor\tIL\tMcLean County\tH1\n61845\t17113\tFoosland\tIL\tMcLean County\tH1\n61738\t17113\tEl paso\tIL\tMcLean County\tH1\n61721\t17113\tArmington\tIL\tMcLean County\tH1\n61731\t17113\tCropsey\tIL\tMcLean County\tH1\n61704\t17113\tBloomington\tIL\tMcLean County\tH1\n61736\t17113\tDowns\tIL\tMcLean County\tH1\n61709\t17113\tBloomington\tIL\tMcLean County\tH1\n62573\t17115\tWarrensburg\tIL\tMacon County\tH1\n62554\t17115\tOreana\tIL\tMacon County\tH1\n62547\t17115\tMount auburn\tIL\tMacon County\tH1\n62549\t17115\tMt zion\tIL\tMacon County\tH1\n62551\t17115\tNiantic\tIL\tMacon County\tH1\n61756\t17115\tMaroa\tIL\tMacon County\tH1\n61937\t17115\tLovington\tIL\tMacon County\tH1\n62537\t17115\tHarristown\tIL\tMacon County\tH1\n61882\t17115\tWeldon\tIL\tMacon County\tH1\n61914\t17115\tBethany\tIL\tMacon County\tH1\n62526\t17115\tDecatur\tIL\tMacon County\tH1\n62539\t17115\tIlliopolis\tIL\tMacon County\tH1\n61925\t17115\tDalton city\tIL\tMacon County\tH1\n62522\t17115\tDecatur\tIL\tMacon County\tH1\n62501\t17115\tArgenta\tIL\tMacon County\tH1\n62523\t17115\tDecatur\tIL\tMacon County\tH1\n61749\t17115\tKenney\tIL\tMacon County\tH1\n62514\t17115\tBoody\tIL\tMacon County\tH1\n62544\t17115\tMacon\tIL\tMacon County\tH1\n62543\t17115\tLatham\tIL\tMacon County\tH1\n62524\t17115\tDecatur\tIL\tMacon County\tH1\n61818\t17115\tCerro gordo\tIL\tMacon County\tH1\n61830\t17115\tCisco\tIL\tMacon County\tH1\n62521\t17115\tDecatur\tIL\tMacon County\tH1\n62513\t17115\tBlue mound\tIL\tMacon County\tH1\n62535\t17115\tForsyth\tIL\tMacon County\tH1\n62550\t17115\tMoweaqua\tIL\tMacon County\tH1\n62525\t17115\tDecatur\tIL\tMacon County\tH1\n62532\t17115\tElwin\tIL\tMacon County\tH1\n62069\t17117\tMount olive\tIL\tMacoupin County\tH1\n62021\t17117\tDorsey\tIL\tMacoupin County\tH1\n62560\t17117\tRaymond\tIL\tMacoupin County\tH1\n62009\t17117\tBenld\tIL\tMacoupin County\tH1\n62056\t17117\tLitchfield\tIL\tMacoupin County\tH1\n62630\t17117\tChesterfield\tIL\tMacoupin County\tH1\n62685\t17117\tShipman\tIL\tMacoupin County\tH1\n62667\t17117\tModesto\tIL\tMacoupin County\tH1\n62012\t17117\tBrighton\tIL\tMacoupin County\tH1\n62674\t17117\tPalmyra\tIL\tMacoupin County\tH1\n62014\t17117\tBunker hill\tIL\tMacoupin County\tH1\n62626\t17117\tCarlinville\tIL\tMacoupin County\tH1\n62672\t17117\tNilwood\tIL\tMacoupin County\tH1\n62033\t17117\tGillespie\tIL\tMacoupin County\tH1\n62088\t17117\tStaunton\tIL\tMacoupin County\tH1\n62097\t17117\tWorden\tIL\tMacoupin County\tH1\n62082\t17117\tRoodhouse\tIL\tMacoupin County\tH1\n62640\t17117\tGirard\tIL\tMacoupin County\tH1\n62079\t17117\tPiasa\tIL\tMacoupin County\tH1\n62091\t17117\tWalshville\tIL\tMacoupin County\tH1\n62638\t17117\tFranklin\tIL\tMacoupin County\tH1\n62093\t17117\tWilsonville\tIL\tMacoupin County\tH1\n62074\t17117\tNew douglas\tIL\tMacoupin County\tH1\n62649\t17117\tHettick\tIL\tMacoupin County\tH1\n62668\t17117\tMurrayville\tIL\tMacoupin County\tH1\n62002\t17117\tAlton\tIL\tMacoupin County\tH1\n62063\t17117\tMedora\tIL\tMacoupin County\tH1\n62044\t17117\tGreenfield\tIL\tMacoupin County\tH1\n62085\t17117\tSawyerville\tIL\tMacoupin County\tH1\n62572\t17117\tWaggoner\tIL\tMacoupin County\tH1\n62690\t17117\tVirden\tIL\tMacoupin County\tH1\n62023\t17117\tEagarville\tIL\tMacoupin County\tH1\n62035\t17119\tGodfrey\tIL\tMadison County\tH1\n62021\t17119\tDorsey\tIL\tMadison County\tH1\n62010\t17119\tBethalto\tIL\tMadison County\tH1\n62025\t17119\tEdwardsville\tIL\tMadison County\tH1\n62060\t17119\tMadison\tIL\tMadison County\tH1\n62249\t17119\tHighland\tIL\tMadison County\tH1\n62275\t17119\tPocahontas\tIL\tMadison County\tH1\n62254\t17119\tLebanon\tIL\tMadison County\tH1\n62048\t17119\tHartford\tIL\tMadison County\tH1\n62084\t17119\tRoxana\tIL\tMadison County\tH1\n62012\t17119\tBrighton\tIL\tMadison County\tH1\n62062\t17119\tMaryville\tIL\tMadison County\tH1\n62201\t17119\tEast saint louis\tIL\tMadison County\tH1\n62001\t17119\tAlhambra\tIL\tMadison County\tH1\n62269\t17119\tO fallon\tIL\tMadison County\tH1\n62058\t17119\tLivingston\tIL\tMadison County\tH1\n62026\t17119\tEdwardsville\tIL\tMadison County\tH1\n62040\t17119\tGranite city\tIL\tMadison County\tH1\n62087\t17119\tSouth roxana\tIL\tMadison County\tH1\n62234\t17119\tCollinsville\tIL\tMadison County\tH1\n62281\t17119\tSaint jacob\tIL\tMadison County\tH1\n62216\t17119\tAviston\tIL\tMadison County\tH1\n62061\t17119\tMarine\tIL\tMadison County\tH1\n62086\t17119\tSorento\tIL\tMadison County\tH1\n62088\t17119\tStaunton\tIL\tMadison County\tH1\n62090\t17119\tVenice\tIL\tMadison County\tH1\n62097\t17119\tWorden\tIL\tMadison County\tH1\n62067\t17119\tMoro\tIL\tMadison County\tH1\n62018\t17119\tCottage hills\tIL\tMadison County\tH1\n62024\t17119\tEast alton\tIL\tMadison County\tH1\n62074\t17119\tNew douglas\tIL\tMadison County\tH1\n62095\t17119\tWood river\tIL\tMadison County\tH1\n62294\t17119\tTroy\tIL\tMadison County\tH1\n62034\t17119\tGlen carbon\tIL\tMadison County\tH1\n62046\t17119\tHamel\tIL\tMadison County\tH1\n62002\t17119\tAlton\tIL\tMadison County\tH1\n62293\t17119\tTrenton\tIL\tMadison County\tH1\n62273\t17119\tPierron\tIL\tMadison County\tH1\n62885\t17121\tShobonier\tIL\tMarion County\tH1\n62892\t17121\tVernon\tIL\tMarion County\tH1\n62899\t17121\tXenia\tIL\tMarion County\tH1\n62882\t17121\tSandoval\tIL\tMarion County\tH1\n62838\t17121\tFarina\tIL\tMarion County\tH1\n62851\t17121\tKeenes\tIL\tMarion County\tH1\n62250\t17121\tHoffman\tIL\tMarion County\tH1\n62807\t17121\tAlma\tIL\tMarion County\tH1\n62830\t17121\tDix\tIL\tMarion County\tH1\n62801\t17121\tCentralia\tIL\tMarion County\tH1\n62875\t17121\tPatoka\tIL\tMarion County\tH1\n62881\t17121\tSalem\tIL\tMarion County\tH1\n62889\t17121\tTexico\tIL\tMarion County\tH1\n62849\t17121\tIuka\tIL\tMarion County\tH1\n62893\t17121\tWalnut hill\tIL\tMarion County\tH1\n62854\t17121\tKinmundy\tIL\tMarion County\tH1\n62853\t17121\tKell\tIL\tMarion County\tH1\n62870\t17121\tOdin\tIL\tMarion County\tH1\n61523\t17123\tChillicothe\tIL\tMarshall County\tH1\n61560\t17123\tPutnam\tIL\tMarshall County\tH1\n61375\t17123\tVarna\tIL\tMarshall County\tH1\n61421\t17123\tBradford\tIL\tMarshall County\tH1\n61358\t17123\tRutland\tIL\tMarshall County\tH1\n61565\t17123\tSparland\tIL\tMarshall County\tH1\n61570\t17123\tWashburn\tIL\tMarshall County\tH1\n61377\t17123\tWenona\tIL\tMarshall County\tH1\n61369\t17123\tToluca\tIL\tMarshall County\tH1\n61424\t17123\tCamp grove\tIL\tMarshall County\tH1\n61526\t17123\tEdelstein\tIL\tMarshall County\tH1\n61537\t17123\tHenry\tIL\tMarshall County\tH1\n61479\t17123\tSpeer\tIL\tMarshall County\tH1\n61336\t17123\tMagnolia\tIL\tMarshall County\tH1\n61541\t17123\tLa rose\tIL\tMarshall County\tH1\n61540\t17123\tLacon\tIL\tMarshall County\tH1\n61321\t17123\tDana\tIL\tMarshall County\tH1\n61760\t17123\tMinonk\tIL\tMarshall County\tH1\n61546\t17125\tManito\tIL\tMason County\tH1\n62627\t17125\tChandlerville\tIL\tMason County\tH1\n62671\t17125\tNew holland\tIL\tMason County\tH1\n62655\t17125\tKilbourne\tIL\tMason County\tH1\n62664\t17125\tMason city\tIL\tMason County\tH1\n62682\t17125\tSan jose\tIL\tMason County\tH1\n61534\t17125\tGreen valley\tIL\tMason County\tH1\n62617\t17125\tBath\tIL\tMason County\tH1\n62644\t17125\tHavana\tIL\tMason County\tH1\n61567\t17125\tTopeka\tIL\tMason County\tH1\n61532\t17125\tForest city\tIL\tMason County\tH1\n62633\t17125\tEaston\tIL\tMason County\tH1\n62960\t17127\tMetropolis\tIL\tMassac County\tH1\n62956\t17127\tKarnak\tIL\tMassac County\tH1\n62943\t17127\tGrantsburg\tIL\tMassac County\tH1\n62938\t17127\tGolconda\tIL\tMassac County\tH1\n62908\t17127\tBelknap\tIL\tMassac County\tH1\n62910\t17127\tBrookport\tIL\tMassac County\tH1\n62941\t17127\tGrand chain\tIL\tMassac County\tH1\n62953\t17127\tJoppa\tIL\tMassac County\tH1\n62625\t17129\tCantrall\tIL\tMenard County\tH1\n62642\t17129\tGreenview\tIL\tMenard County\tH1\n62688\t17129\tTallula\tIL\tMenard County\tH1\n62659\t17129\tLincolns new salem\tIL\tMenard County\tH1\n62693\t17129\tWilliamsville\tIL\tMenard County\tH1\n62613\t17129\tAthens\tIL\tMenard County\tH1\n62666\t17129\tMiddletown\tIL\tMenard County\tH1\n62673\t17129\tOakford\tIL\tMenard County\tH1\n62675\t17129\tPetersburg\tIL\tMenard County\tH1\n61412\t17131\tAlexis\tIL\tMercer County\tH1\n61486\t17131\tViola\tIL\tMercer County\tH1\n61272\t17131\tNew boston\tIL\tMercer County\tH1\n61263\t17131\tMatherville\tIL\tMercer County\tH1\n61401\t17131\tGalesburg\tIL\tMercer County\tH1\n61465\t17131\tNew windsor\tIL\tMercer
